vi "FTW-Container-Element-Set.vi"(0 "FTW-Container In":refnum<class "FTW-Container.lvclass">, 5 "Element Name":string, 7 "Value":variant, 11 "error in":errorcluster) -> (4 "FTW-Container Out":refnum<class "FTW-Container.lvclass">, 8 "Replaced":bool, 15 "error out":errorcluster)   [LabVIEW 2015, in "FTW-Container.lvclass"]
uses:
  FTW-Container.lvclass
  FTW-Container.lvclass/FTW-Container.ctl
  <vilib>/Utility/Data Type/NI_Data Type.lvlib
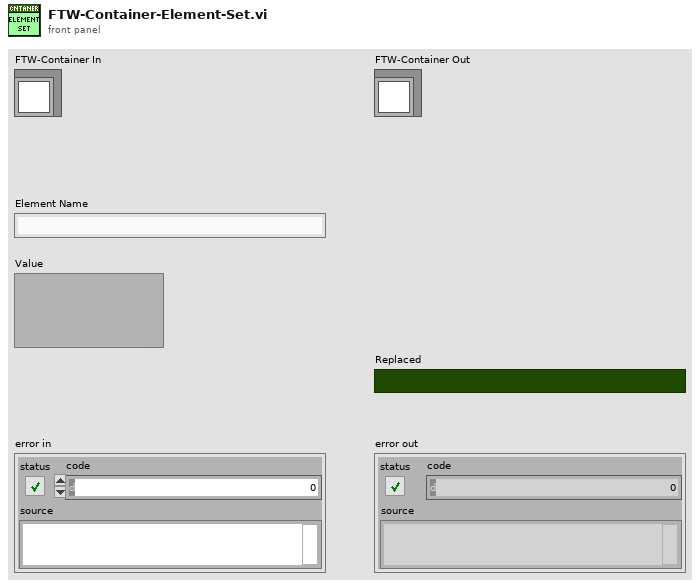
[diagram p1: front panel]
types:
  T1 = typedef "NI_Data Type.lvlib/Data Type.ctl" = enum8{"Invalid Type", "Void", "I8", "I16", "I32", "I64", "U8", "U16", "U32", "U64", "Single Float", "Double Float", "Extended Float", "Single Complex", "Double Complex", "Extended Complex", "Enum U8", "Enum U16", "Enum U32", "Enum U64", "Single Float With Unit", "Double Float With Unit", "Extended Float With Unit", "Single Complex with Unit", "Double Complex with Unit", "Extended Complex with Unit", "Boolean", "String", "Path", "Picture", "Tag", "Array", "Cluster", "Variant", "LV Variant", "Waveform", "Timestamp", "Digital Waveform", "Digital Data", "ExpressData", "Refnum", "External Data", "VI", "Poly VI", "LabVIEW Class Instance", "Fixed Point"}
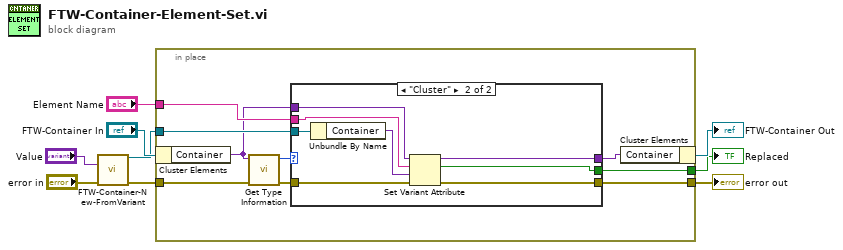
[diagram p0: block diagram]
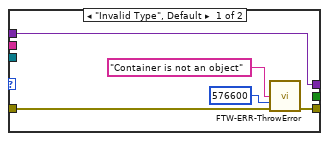
[diagram p2: hidden frame]
diagram:
  n1 = call "FTW-Container-New-FromVariant.vi"("Variant"="Value", "error in"="error in") -> ("FTW-Container"=w1:refnum<class "FTW-Container.lvclass">, "error out"=w3:errorcluster)  [unwired: 12 in]
  n2 = in-place {
    in-place-border: [w17] -> w7
    in-place-border: w3 -> [w18]
    in-place-border: "Element Name" -> [w15]
    in-place-border: w1 -> [w12]
    in-place-border: [w10] -> w4
    n3 = in-place-cluster #1("FTW-Container In") -> ("Container"=w11:variant)
    n4 = call <vilib>:"Get Type Information.vi"("error in (no error)"=w18, "Variant"=w11) -> ("error out"=w14:errorcluster, "Type"=w13:T1)  [unwired: 5 in, 3 out]
    n5 = case shown="\"Cluster\"" w13 {
      tunnel: w14 -> [w21 w31]
      tunnel: [w20 w30] -> w17
      tunnel: w11 -> [w19 w29]
      tunnel: [w19 w26] -> w16
      tunnel: w15 -> [_ w27]
      tunnel: w12 -> [_ w28]
      tunnel: [_ w25] -> w10
      frame "Invalid Type", Default {
        n6 = call "FTW-ERR-ThrowError.vi"("Error Message"="Container is not an object", "Error Code"=576600, "error in"=w21) -> ("error out"=w20:errorcluster)  [unwired: 12 in]
      }
      frame "Cluster" {
        n7 = Unbundle By Name(w28) -> ("Container"=w24:variant)
        n8 = Set Variant Attribute(Variant=w29, name=w27, value=w24, error in=w31) -> (Variant out=w26:variant, replaced=w25:bool, error out=w30:errorcluster)
      }
    }
    n9 = in-place-cluster #1("Container"=w16) -> (→"FTW-Container Out":refnum<class "FTW-Container.lvclass">)
  }
  "error out" <- w7
  "Replaced" <- w4
